vi "GetDeviceConfig.vi"(8 "error in (no error)":errorcluster, 11 "Device":T1) -> (0 "error out":errorcluster, 1 "Sample Rate":dbl, 2 "Number of Dynamic Modules":i32, 3 "Name":string)   [LabVIEW 2015]
uses:
  <vilib>/addons/InsightCM/MessageBus/Base/controls/Device.ctl
  <vilib>/addons/InsightCM/MessageBus/Base/controls/KeyValuePair.ctl
  <vilib>/addons/InsightCM/MessageBus/Base/controls/DataGroup.ctl
  <vilib>/addons/InsightCM/MessageBus/Base/controls/OperatingState.ctl
  <vilib>/addons/InsightCM/MessageBus/Base/controls/Trigger.ctl
  <vilib>/addons/InsightCM/MessageBus/Base/controls/Condition.ctl
  <vilib>/addons/InsightCM/Utilities/PropertyHelpers/PropertyHelpers.lvlib
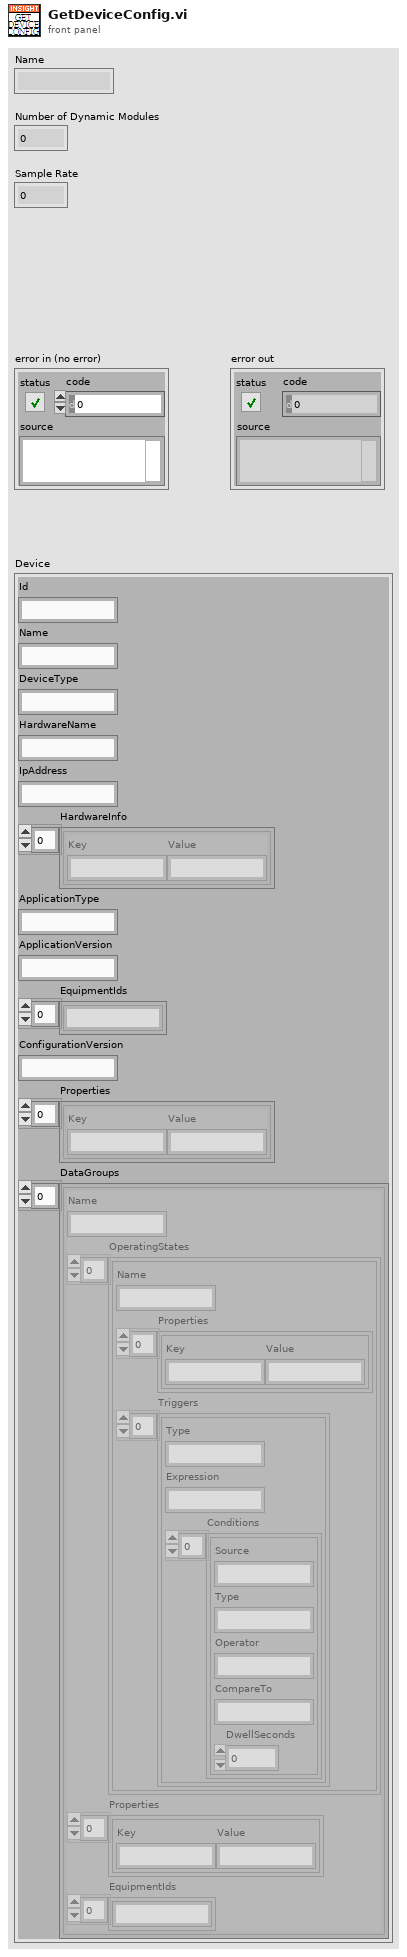
[diagram p1: front panel]
types:
  T1 = typedef "Device.ctl" = cluster{"Id":string, "Name":string, "DeviceType":string, "HardwareName":string, "IpAddress":string, "HardwareInfo":T2[], "ApplicationType":string, "ApplicationVersion":string, "EquipmentIds":string[], "ConfigurationVersion":string, "Properties":T2[], "DataGroups":T3[]}
  T2 = typedef "KeyValuePair.ctl" = cluster{"Key":string, "Value":string}
  T3 = typedef "DataGroup.ctl" = cluster{"Name":string, "OperatingStates":T4[], "Properties":T2[], "EquipmentIds":string[]}
  T4 = typedef "OperatingState.ctl" = cluster{"Name":string, "Properties":T2[], "Triggers":T5[]}
  T5 = typedef "Trigger.ctl" = cluster{"Type":string, "Expression":string, "Conditions":T6[]}
  T6 = typedef "Condition.ctl" = cluster{"Source":string, "Type":string, "Operator":string, "CompareTo":string, "DwellSeconds":dbl}
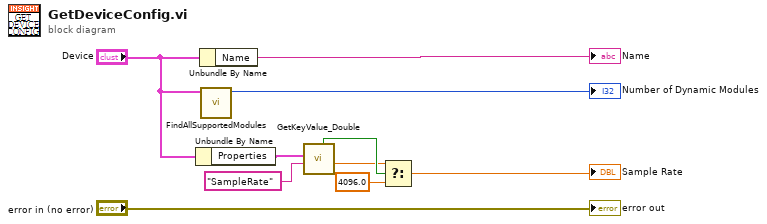
[diagram p0: block diagram]
diagram:
  n1 = Unbundle By Name("Device") -> ("Properties"=w3:T2[])
  n2 = Unbundle By Name("Device") -> ("Name"=→"Name":string)
  n3 = call "FindAllSupportedModules.vi"("Device Model"="Device") -> ("Number of Supported Modules"=→"Number of Dynamic Modules":i32)  [unwired: 9 in, 1 out]
  n4 = call <vilib>:"GetKeyValue_Double.vi"("key"="SampleRate", "key value pairs"=w3) -> ("value"=w1:dbl, "found"=w6:bool)  [unwired: 7 in, 1 out]
  n5 = Select(t=w1, s=w6, f=4096.0) -> (s? t:f=→"Sample Rate":dbl)
  "error out" <- "error in (no error)"
